vi "dfd_Classify Roots.vi"(11 "Roots":cdb[](array[numeric])) -> (0 "# zero-inf root":i32, 2 "real roots":dbl[](array[numeric]) format="%#_6e", 3 "conj roots":cdb[](array[numeric]))   [LabVIEW 2017, in "NI_DigFilterLicensed.lvlib"]
uses:
  <vilib>/addons/Digital Filter Design/NI_DigFilterLicensed.lvlib
  <vilib>/Analysis/polynomials.llb/Polynomial Roots (DBL).vi
  <vilib>/Analysis/polynomials.llb/Create Polynomial From Roots (CDB).vi
  <vilib>/Analysis/NI_AALPro.lvlib
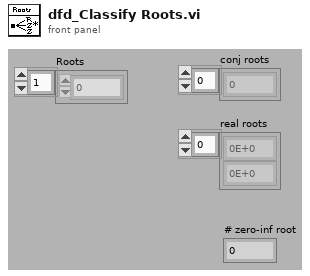
[diagram p1: front panel]
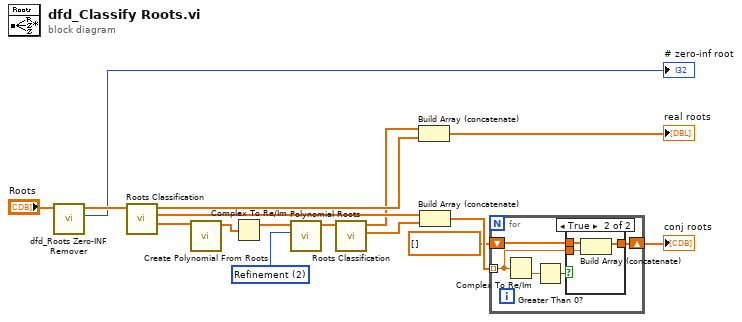
[diagram p0: block diagram]
diagram:
  w1 = u16 2 items=["General", "Simple Classification", "Refinement", "Advanced Refinement"] ("option")
  n1 = call <vilib>:"dfd_Roots Zero-INF Remover.vi"("roots"="Roots") -> ("# zero root"=→"# zero-inf root":i32, "new roots"=w4:cdb[])  [unwired: 9 out]
  n2 = call <vilib>:"Roots Classification.vi"("Roots"=w4) -> ("Pure Complex Roots"=w11:cdb[], "Complex Pair Roots"=w13:cdb[], "Real Roots"=w12:dbl[])  [unwired: 2 in, 6 out]
  n3 = call-poly <vilib>:"Create Polynomial From Roots.vi"("Roots"=w11) -> ("P(x)"=w10:cdb[])  [unwired: 10 out]
  n4 = Complex To Re/Im(x + iy=w10) -> (x=w5:dbl[])  [unwired: 1 out]
  n5 = call-poly <vilib>:"Polynomial Roots.vi"("option"=w1, "P(x)"=w5) -> ("Roots"=w9:cdb[])  [unwired: 9 out]
  n6 = call <vilib>:"Roots Classification.vi"("Roots"=w9) -> ("Complex Pair Roots"=w7:cdb[], "Real Roots"=w8:dbl[])  [unwired: 2 in, 7 out]
  n7 = Build Array (concatenate)(w8, w12) -> (→"real roots":dbl[])
  n8 = Build Array (concatenate)(w13, w7) -> (w15:cdb[])
  n9 = for {
    tunnel: w15 -> [w19] mode=indexing
    shift-right: [w20] -> w16
    shift-left: cdb[] [] -> [w18]
    n10 = Complex To Re/Im(x + iy=w19) -> (y=w21:dbl)  [unwired: 1 out]
    n11 = Greater Than 0?(x=w21) -> (x > 0?=w17:bool)
    n12 = case shown="True" w17 {
      tunnel: [w22 w25] -> w20
      tunnel: w19 -> [_ w24]
      tunnel: w18 -> [w22 w23]
      frame False {
      }
      frame True {
        n13 = Build Array (concatenate)(w23, w24) -> (w25:cdb[])
      }
    }
  }
  "conj roots" <- w16
